vi "EventStruct.vi"() -> ()   [LabVIEW 2021]
panel:
  out "Contador de pulsos":dbl
  in  "Up Button":bool
  in  "Down Button":bool
  out "TIMEOUT":i32
  out "LED":bool
  in  "BOTON 1":bool
  out "I":i32
  in  "stop":bool
  # "Mendoza Meza Manuel Everardo"
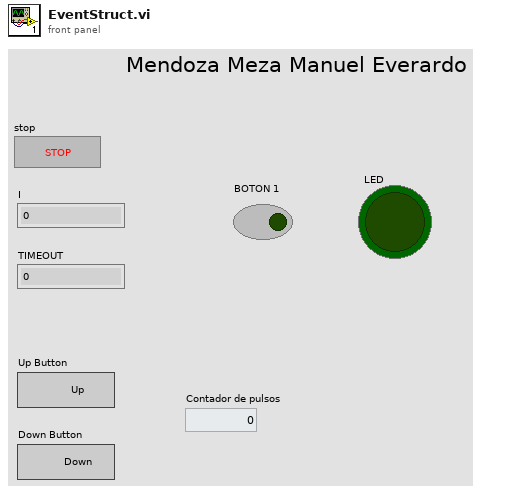
[diagram p1: front panel]
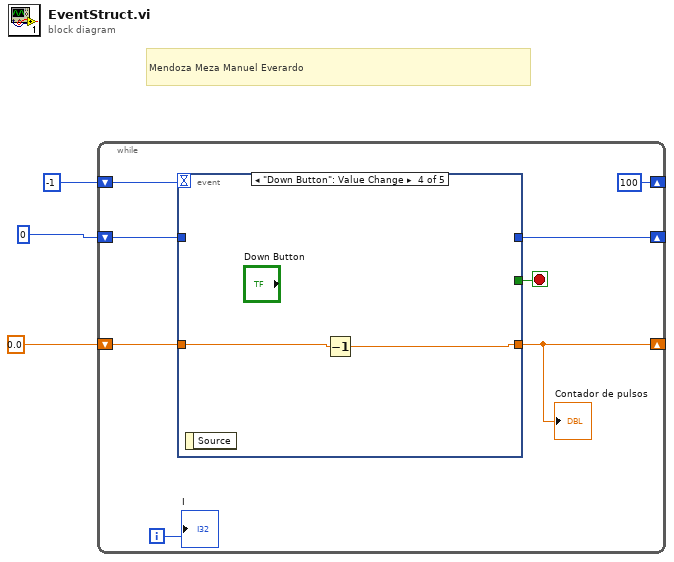
[diagram p0: block diagram]
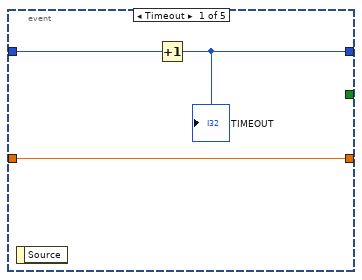
[diagram p2: hidden frame]
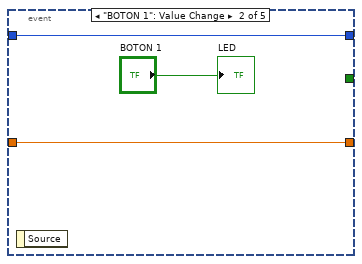
[diagram p3: hidden frame]
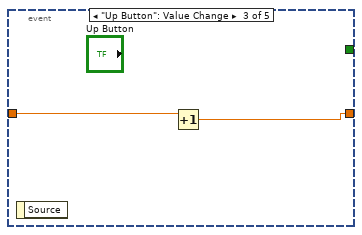
[diagram p4: hidden frame]
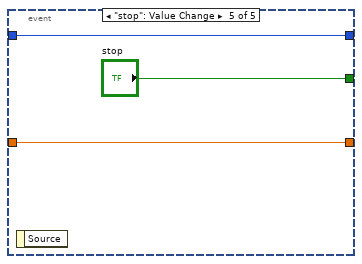
[diagram p5: hidden frame]
diagram:
  # "Mendoza Meza Manuel Everardo"
  n1 = while {
    shift-right: [w8] -> _
    shift-left: 0 -> [w9]
    shift-right: [w6] -> _
    shift-left: 0.0 -> [w7]
    shift-right: [100] -> _
    shift-left: -1 -> [w5]
    i -> [w11]
    stop <- w10 stop-if-true
    n2 = event shown="[3] \"Down Button\": Value Change" {
      selector: _ -> [_ _ _ _ _]
      dyn-events: _ -> [_ _ _ _ _]
      timeout: w5 -> [_ _ _ _ _]
      tunnel: [_ _ _ _ "stop"] -> w10
      tunnel: w9 -> [w14 w16 _ _ w23]
      tunnel: [w13 w16 _ _ w23] -> w8
      tunnel: w7 -> [w12 w15 w19 w21 w22]
      tunnel: [w12 w15 w18 w20 w22] -> w6
      event Timeout {
        n3 = event-data() -> ()  [unwired: 1 in, 1 out]
        n4 = Increment(x=w14) -> (x+1=w13:i32)
        "TIMEOUT" <- w13
      }
      event "BOTON 1": Value Change {
        n5 = event-data() -> ()  [unwired: 1 in, 1 out]
        "LED" <- "BOTON 1"
      }
      event "Up Button": Value Change {
        n6 = event-data() -> ()  [unwired: 1 in, 1 out]
        n7 = Increment(x=w19) -> (x+1=w18:dbl)
      }
      event "Down Button": Value Change {
        n8 = event-data() -> ()  [unwired: 1 in, 1 out]
        n9 = Decrement(x=w21) -> (x-1=w20:dbl)
      }
      event "stop": Value Change {
        n10 = event-data() -> ()  [unwired: 1 in, 1 out]
      }
    }
    "Contador de pulsos" <- w6
    "I" <- w11
  }
